vi "angleBetweenRobotDest.vi"(8 "error in (no error)":errorcluster, 9 "dest(i+1) - dest(i)":dbl[](array[numeric]), 10 "dest(i) - robot":dbl[](array[numeric]), 11 "Game in":refnum<class "Game.lvclass">) -> (0 "error out":errorcluster, 2 "halfAngleBetweenVectors":dbl, 3 "Game out":refnum<class "Game.lvclass">)   [LabVIEW 2023, in "Game.lvclass"]
uses:
  Game.lvclass
  Utilities_class/Utilities.lvclass
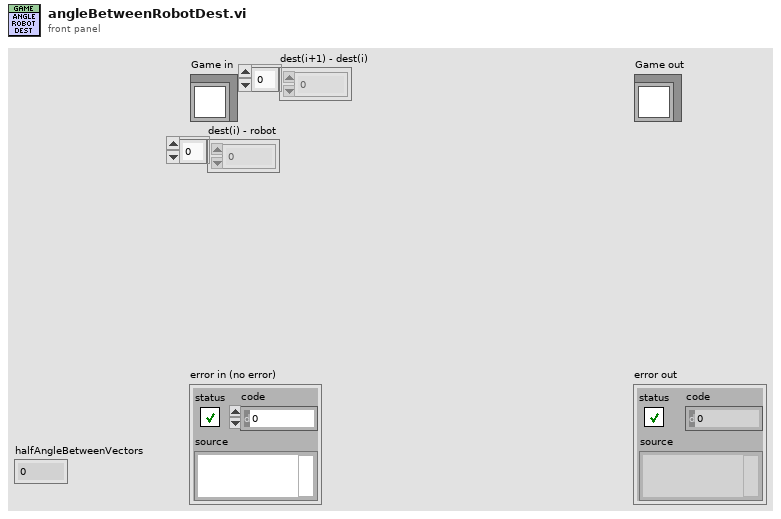
[diagram p1: front panel]
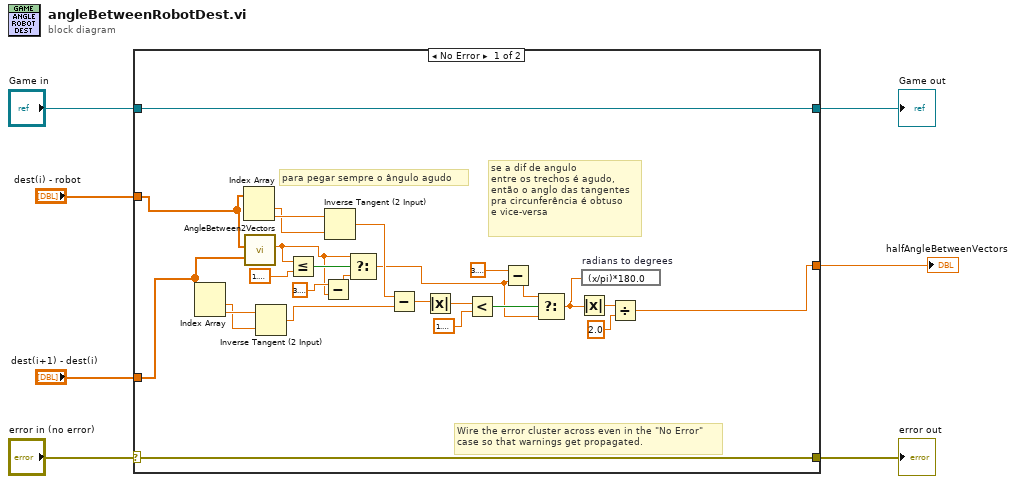
[diagram p0: block diagram]
diagram:
  n1 = case shown="No Error" "error in (no error)" {
    selector: "error in (no error)" -> [w32 w35]
    tunnel: [w32 w35] -> w6
    tunnel: [w33 w34] -> w4
    tunnel: "Game in" -> [w33 w34]
    tunnel: "dest(i) - robot" -> [w10 _]
    tunnel: "dest(i+1) - dest(i)" -> [w9 _]
    tunnel: [w8 _] -> w1
    frame No Error {
      # "se a dif de angulo\nentre os trechos é agudo,\nentão o anglo das tangentes\npra circunferência é obtuso\ne vice-versa"
      # "para pegar sempre o ângulo agudo"
      # "Wire the error cluster across even in the \"No Error\"\ncase so that warnings get propagated."
      n2 = Index Array(array=w9) -> (element #1=w28:dbl, element #2=w29:dbl)  [unwired: 2 in]
      n3 = Index Array(array=w10) -> (element #1=w30:dbl, element #2=w31:dbl)  [unwired: 2 in]
      n4 = call "AngleBetween2Vectors.vi"("Array 1"=w9, "Array 2"=w10) -> ("angleInRadians(default)"=w12:dbl)  [unwired: 6 in, 3 out]
      n5 = Inverse Tangent (2 Input)(1:w28, 2:w29) -> (0:w26:dbl)
      n6 = Less Or Equal?(x=w12, y=1.5707963267948966) -> (x <= y?=w15:bool)
      n7 = Subtract(x=3.141592653589793, y=w12) -> (x-y=w13:dbl)
      n8 = Inverse Tangent (2 Input)(1:w30, 2:w31) -> (0:w27:dbl)
      n9 = Select(t=w12, s=w15, f=w13) -> (s? t:f=w11:dbl)
      n10 = Subtract(x=w27, y=w26) -> (x-y=w25:dbl)
      n11 = Absolute Value(x=w25) -> (abs(x)=w24:dbl)
      n12 = Less?(x=w24, y=1.5707963267948966) -> (x < y?=w22:bool)
      n13 = Subtract(x=3.141592653589793, y=w11) -> (x-y=w20:dbl)
      n14 = Select(t=w20, s=w22, f=w11) -> (s? t:f=w19:dbl)
      n15 = Absolute Value(x=w19) -> (abs(x)=w18:dbl)
      n16 = expression code="(x/pi)*180.0" "radians to degrees"(w19) -> ()  [unwired: 1 out]
      n17 = Divide(x=w18, y=2.0) -> (x/y=w8:dbl)
    }
    frame Error {
    }
  }
  "error out" <- w6
  "Game out" <- w4
  "halfAngleBetweenVectors" <- w1
